vi "check if user is admin.vi"(11 "username":string) -> (2 "user is admin":bool)   [LabVIEW 2024]
uses:
  CTRLS/DB operation Selector.ctl
panel:
  out "error out":errorcluster
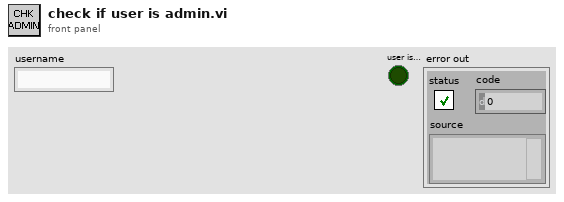
[diagram p1: front panel]
types:
  T1 = typedef "DB operation Selector.ctl" = enum16{"Select", "Insert", "Update", "Execute select Query", "Execute update query"}
  T2 = typedef "NI_Database_API.lvlib/Conn ObjectReference.ctl" = refnum<k1>
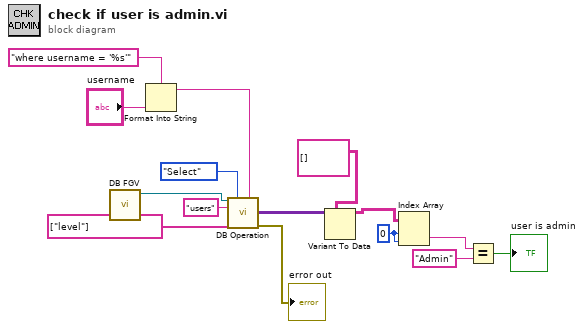
[diagram p0: block diagram]
diagram:
  w5 = 0 ("index (row)")
  n1 = call "DB FGV.vi"() -> ("DB ref"=w9:T2)  [unwired: 11 in]
  n2 = Format Into String(format string="where username = '%s'", "username") -> (resulting string=w10:string)  [unwired: 2 in, 1 out]
  n3 = call "DB Operation.vi"("connection reference"=w9, "DB Op Selector"=DB_operation_Selector."Select", "Condition"=w10, "table"="users", "columns"=string[] ["level"]) -> ("data out"=w7:variant[][], "error out"=→"error out":errorcluster)  [unwired: 8 in, 1 out]
  n4 = Variant To Data(type=string[][] [] ("columns"), Variant=w7) -> (data=w6:string[][])  [unwired: 1 in, 1 out]
  n5 = Index Array(array=w6, index (row)=w5, index (col)=w5) -> (element=w4:string)
  n6 = Equal?(x=w4, y="Admin") -> (x = y?=→"user is admin":bool)
